vi "RSZVB Set Calibration Correction Base Frequency State.vi"(8 "error in (no error)":errorcluster {"code" format="%.0x"}, 9 "State (F: Off)":bool, 10 "Channel (1)":i32=1, 11 "VISA session":refnum<visa-resource-name>) -> (0 "error out":errorcluster {"code" format="%.0x"}, 3 "dup VISA session":refnum<visa-resource-name>)   [LabVIEW 2011]
doc: "This VI force calibration and system error correction to be performed at base frequency for setups with external frequency conversion.\n\nRemote-control command(s):ee\n[SENSe<Ch>:]CORRection:CBFReq[:STATe]"
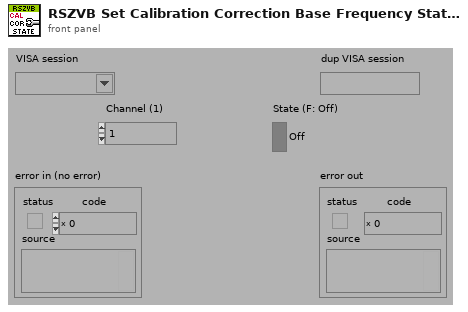
[diagram p1: front panel]
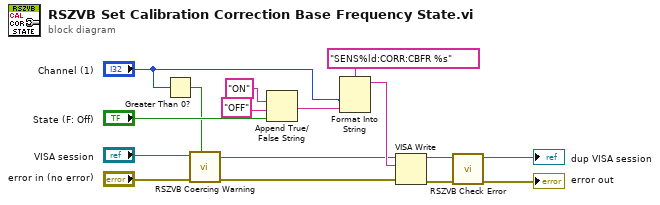
[diagram p0: block diagram]
diagram:
  n1 = Greater Than 0?(x="Channel (1)") -> (x > 0?=w8:bool)
  n2 = call "RSZVB Coercing Warning.vi"("In Range?"=w8, "error in (no error)"="error in (no error)", "VISA session"="VISA session") -> ("error out"=w4:errorcluster, "dup VISA session"=w3:refnum<visa-resource-name>)  [unwired: 7 in]
  n3 = Append True/False String(1:"State (F: Off)", 2:"OFF", 3:"ON") -> (0:w9:string)  [unwired: 1 in]
  n4 = Format Into String(format string="SENS%ld:CORR:CBFR %s", "Channel (1)", w9) -> (resulting string=w13:string)  [unwired: 2 in, 1 out]
  n5 = VISA Write(VISA resource name=w3, write buffer=w13, error in (no error)=w4) -> (VISA resource name out=w14:refnum<visa-resource-name>, error out=w15:errorcluster)  [unwired: 1 out]
  n6 = call "RSZVB Check Error.vi"("error in (no error)"=w15, "VISA session"=w14) -> ("error out"=→"error out":errorcluster, "dup VISA session"=→"dup VISA session":refnum<visa-resource-name>)  [unwired: 8 in]
